vi "tm_preparecapture.vi"(8 "error in (no error)":errorcluster {"code" format="%.0x"}, 9 "Frames":i32, 10 "Capture mode":i32(ring) items=["Snap", "Sequence"], 11 "Handle in":u32) -> (0 "error out":errorcluster {"code" format="%.0x"}, 2 "Buffer Info":T1, 3 "Handle out":u32, 4 "Image type":u32)   [LabVIEW 2017]
uses:
  tmcamcon.dll
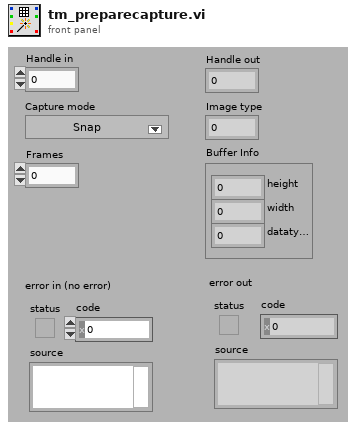
[diagram p1: front panel]
types:
  T1 = cluster{"height":u32, "width":u32, "datatype":u32}
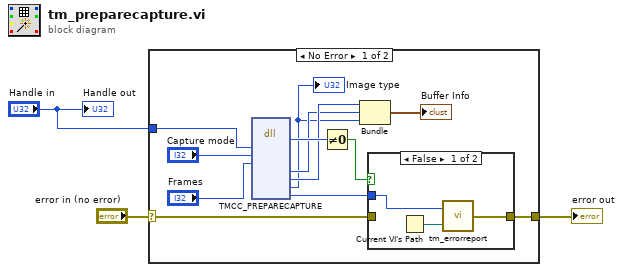
[diagram p0: block diagram]
diagram:
  n1 = case shown="No Error" "error in (no error)" {
    selector: "error in (no error)" -> [w7 w20]
    tunnel: [w4 w20] -> w1
    tunnel: "Handle in" -> [w14 _]
    frame No Error {
      n2 = dll-call lib="tmcamcon.dll" fn="TMCC_PREPARECAPTURE"("index"=w14, "mode"="Capture mode", "frames"="Frames") -> ("return type"=w15:u32, "width"=w10:u32, "height"=w11:u32, "datatype"=w9:u32, "Erval"=w6:i32)  [unwired: 10 in, 2 out]
      "Image type" <- w9
      n3 = Not Equal To 0?(x=w15) -> (x != 0?=w5:bool)
      n4 = Bundle("height"=w11, "width"=w10, "datatype"=w9) -> (→"Buffer Info":T1)  [unwired: 1 in]
      n5 = case shown="False" w5 {
        tunnel: w7 -> [_ w19]
        tunnel: [w16 w19] -> w4
        tunnel: w6 -> [w17 _]
        frame False {
          n6 = Current VI's Path() -> (path=w18:path)
          n7 = call "tm_errorreport.vi"("Source"=w18, "Error"=w17) -> ("error out"=w16:errorcluster)
        }
        frame True {
        }
      }
    }
    frame Error {
    }
  }
  "error out" <- w1
  "Handle out" <- "Handle in"
